vi "Grobal Var Initialize.vi"(8 "에러 입력":errorcluster caption="에러 입력(에러 없음)", 11 "Func_ext":string) -> (0 "에러 출력":errorcluster)   [LabVIEW 2020]
uses:
  Controls/Cmd_Var Data IO.ctl
  Variables/Global_Cal Info.vi
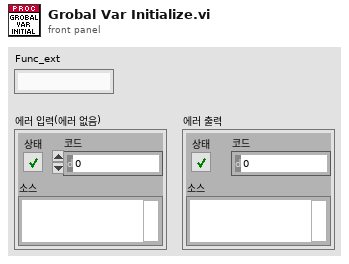
[diagram p1: front panel]
types:
  T1 = typedef "Cmd_Var Data IO.ctl" = enum16{"Condition", "Condition Default", "Condition_Temp", "Resolution", "Resolution Default", "Resolution Old", "Spec", "Spec Default", "Spec Old", "Spec Temp", "Result", "Result2", "Result3", "Result_Temp", "Result_ADJ", "Result_ADJ2", "STD1", "STD2", "STD3", "STD4", "STD5", "STD Temp", "CMC", "CMC Default"}
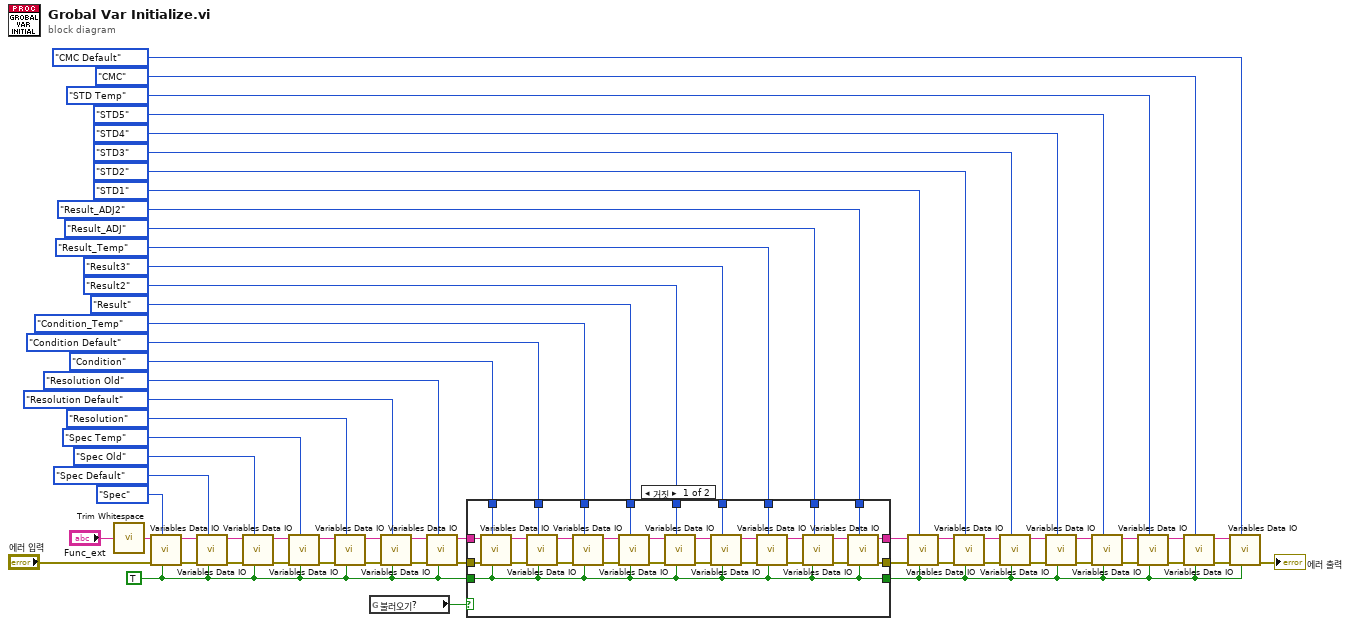
[diagram p0: block diagram]
diagram:
  w8 = TRUE ("Write blank data ?(T)")
  n1 = call <vilib>:"Trim Whitespace.vi"("string"="Func_ext") -> ("trimmed string"=w9:string)  [unwired: 1 in]
  n2 = call "Variables Data IO.vi"("Write blank data ?(F)"=w8, "Select"=Cmd_Var_Data_IO."Spec", "error in"="에러 입력", "Func_ext"=w9) -> ("error out"=w44:errorcluster, "Func_ext Out"=w24:string)  [unwired: 5 in, 1 out]
  n3 = call "Variables Data IO.vi"("Write blank data ?(F)"=w8, "Select"=Cmd_Var_Data_IO."Spec Default", "error in"=w44, "Func_ext"=w24) -> ("error out"=w43:errorcluster, "Func_ext Out"=w23:string)  [unwired: 5 in, 1 out]
  n4 = call "Variables Data IO.vi"("Write blank data ?(F)"=w8, "Select"=Cmd_Var_Data_IO."Spec Old", "error in"=w43, "Func_ext"=w23) -> ("error out"=w42:errorcluster, "Func_ext Out"=w22:string)  [unwired: 5 in, 1 out]
  n5 = call "Variables Data IO.vi"("Write blank data ?(F)"=w8, "Select"=Cmd_Var_Data_IO."Spec Temp", "error in"=w42, "Func_ext"=w22) -> ("error out"=w41:errorcluster, "Func_ext Out"=w21:string)  [unwired: 5 in, 1 out]
  n6 = call "Variables Data IO.vi"("Write blank data ?(F)"=w8, "Select"=Cmd_Var_Data_IO."Resolution", "error in"=w41, "Func_ext"=w21) -> ("error out"=w40:errorcluster, "Func_ext Out"=w20:string)  [unwired: 5 in, 1 out]
  n7 = global read "Global_Cal Info.vi" "불러오기?"() -> (w6:bool)
  n8 = call "Variables Data IO.vi"("Write blank data ?(F)"=w8, "Select"=Cmd_Var_Data_IO."Resolution Default", "error in"=w40, "Func_ext"=w20) -> ("error out"=w39:errorcluster, "Func_ext Out"=w19:string)  [unwired: 5 in, 1 out]
  n9 = call "Variables Data IO.vi"("Write blank data ?(F)"=w8, "Select"=Cmd_Var_Data_IO."Resolution Old", "error in"=w39, "Func_ext"=w19) -> ("error out"=w38:errorcluster, "Func_ext Out"=w18:string)  [unwired: 5 in, 1 out]
  n10 = case shown="거짓" w6 {
    tunnel: Cmd_Var_Data_IO."Condition" ("Select") -> [w91 _]
    tunnel: Cmd_Var_Data_IO."Condition Default" ("Select") -> [w90 _]
    tunnel: Cmd_Var_Data_IO."Result" ("Select") -> [w89 _]
    tunnel: Cmd_Var_Data_IO."Result2" ("Select") -> [w88 _]
    tunnel: Cmd_Var_Data_IO."Result_Temp" ("Select") -> [w87 _]
    tunnel: w38 -> [w86 w93]
    tunnel: [w64 w93] -> w37
    tunnel: Cmd_Var_Data_IO."Result3" ("Select") -> [w84 _]
    tunnel: w18 -> [w83 w94]
    tunnel: [w65 w94] -> w17
    tunnel: w8 -> [w63 w92]
    tunnel: Cmd_Var_Data_IO."Condition_Temp" ("Select") -> [w77 _]
    tunnel: [w63 w92] -> w5
    tunnel: Cmd_Var_Data_IO."Result_ADJ" ("Select") -> [w68 _]
    tunnel: Cmd_Var_Data_IO."Result_ADJ2" ("Select") -> [w62 _]
    frame False {
      n11 = call "Variables Data IO.vi"("Write blank data ?(F)"=w63, "Select"=w91, "error in"=w86, "Func_ext"=w83) -> ("error out"=w85:errorcluster, "Func_ext Out"=w82:string)  [unwired: 5 in, 1 out]
      n12 = call "Variables Data IO.vi"("Write blank data ?(F)"=w63, "Select"=w90, "error in"=w85, "Func_ext"=w82) -> ("error out"=w81:errorcluster, "Func_ext Out"=w80:string)  [unwired: 5 in, 1 out]
      n13 = call "Variables Data IO.vi"("Write blank data ?(F)"=w63, "Select"=w77, "error in"=w81, "Func_ext"=w80) -> ("error out"=w79:errorcluster, "Func_ext Out"=w78:string)  [unwired: 5 in, 1 out]
      n14 = call "Variables Data IO.vi"("Write blank data ?(F)"=w63, "Select"=w89, "error in"=w79, "Func_ext"=w78) -> ("error out"=w76:errorcluster, "Func_ext Out"=w73:string)  [unwired: 5 in, 1 out]
      n15 = call "Variables Data IO.vi"("Write blank data ?(F)"=w63, "Select"=w88, "error in"=w76, "Func_ext"=w73) -> ("error out"=w75:errorcluster, "Func_ext Out"=w72:string)  [unwired: 5 in, 1 out]
      n16 = call "Variables Data IO.vi"("Write blank data ?(F)"=w63, "Select"=w84, "error in"=w75, "Func_ext"=w72) -> ("error out"=w74:errorcluster, "Func_ext Out"=w71:string)  [unwired: 5 in, 1 out]
      n17 = call "Variables Data IO.vi"("Write blank data ?(F)"=w63, "Select"=w87, "error in"=w74, "Func_ext"=w71) -> ("error out"=w69:errorcluster, "Func_ext Out"=w70:string)  [unwired: 5 in, 1 out]
      n18 = call "Variables Data IO.vi"("Write blank data ?(F)"=w63, "Select"=w68, "error in"=w69, "Func_ext"=w70) -> ("error out"=w67:errorcluster, "Func_ext Out"=w66:string)  [unwired: 5 in, 1 out]
      n19 = call "Variables Data IO.vi"("Write blank data ?(F)"=w63, "Select"=w62, "error in"=w67, "Func_ext"=w66) -> ("error out"=w64:errorcluster, "Func_ext Out"=w65:string)  [unwired: 5 in, 1 out]
    }
    frame True {
    }
  }
  n20 = call "Variables Data IO.vi"("Write blank data ?(F)"=w5, "Select"=Cmd_Var_Data_IO."STD1", "error in"=w37, "Func_ext"=w17) -> ("error out"=w36:errorcluster, "Func_ext Out"=w16:string)  [unwired: 5 in, 1 out]
  n21 = call "Variables Data IO.vi"("Write blank data ?(F)"=w5, "Select"=Cmd_Var_Data_IO."STD2", "error in"=w36, "Func_ext"=w16) -> ("error out"=w30:errorcluster, "Func_ext Out"=w15:string)  [unwired: 5 in, 1 out]
  n22 = call "Variables Data IO.vi"("Write blank data ?(F)"=w5, "Select"=Cmd_Var_Data_IO."STD3", "error in"=w30, "Func_ext"=w15) -> ("error out"=w29:errorcluster, "Func_ext Out"=w14:string)  [unwired: 5 in, 1 out]
  n23 = call "Variables Data IO.vi"("Write blank data ?(F)"=w5, "Select"=Cmd_Var_Data_IO."STD4", "error in"=w29, "Func_ext"=w14) -> ("error out"=w28:errorcluster, "Func_ext Out"=w13:string)  [unwired: 5 in, 1 out]
  n24 = call "Variables Data IO.vi"("Write blank data ?(F)"=w5, "Select"=Cmd_Var_Data_IO."STD5", "error in"=w28, "Func_ext"=w13) -> ("error out"=w27:errorcluster, "Func_ext Out"=w12:string)  [unwired: 5 in, 1 out]
  n25 = call "Variables Data IO.vi"("Write blank data ?(F)"=w5, "Select"=Cmd_Var_Data_IO."STD Temp", "error in"=w27, "Func_ext"=w12) -> ("error out"=w35:errorcluster, "Func_ext Out"=w11:string)  [unwired: 5 in, 1 out]
  n26 = call "Variables Data IO.vi"("Write blank data ?(F)"=w5, "Select"=Cmd_Var_Data_IO."CMC", "error in"=w35, "Func_ext"=w11) -> ("error out"=w34:errorcluster, "Func_ext Out"=w10:string)  [unwired: 5 in, 1 out]
  n27 = call "Variables Data IO.vi"("Write blank data ?(F)"=w5, "Select"=Cmd_Var_Data_IO."CMC Default", "error in"=w34, "Func_ext"=w10) -> ("error out"=→"에러 출력":errorcluster)  [unwired: 5 in, 2 out]
